vi "Add form to database.vi"(7 "Name":string, 8 "error in (no error)":errorcluster, 11 "Form Server Wrapper in":refnum<class "Form Server Wrapper.lvclass">) -> (0 "error out":errorcluster, 3 "Form Server Wrapper out":refnum<class "Form Server Wrapper.lvclass">)   [LabVIEW 2020, in "Form Server.lvlib" / "Form Server Wrapper.lvclass"]
uses:
  Form Server Wrapper.lvclass
  Form Server Wrapper.lvclass/Form Server Wrapper.ctl
  Form Server Messages Messages/Add Row to Database Msg/Add Row to Database Msg.lvclass/Add Row to Database Msg.ctl
  <vilib>/ActorFramework/Message Enqueuer/Message Enqueuer.lvclass/Message Enqueuer.ctl
  <vilib>/ActorFramework/Message Enqueuer/Enqueue.vi
  Form Server Messages Messages/Add Row to Database Msg/Add Row to Database Msg.lvclass
  C:/Program Files (x86)/National Instruments/LabVIEW 2020/vi.lib/ActorFramework/Message/Message.lvclass
  <vilib>/ActorFramework/Message Priority Queue/Priority Enqueue.vi
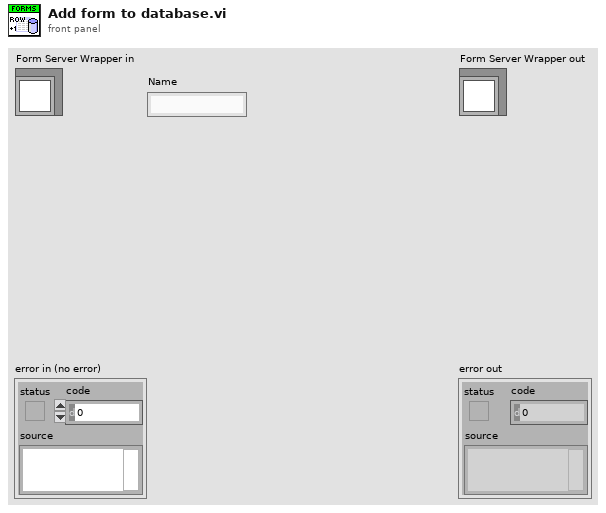
[diagram p1: front panel]
types:
  T1 = typedef "Form Server Interfaces.lvlib/Form ID.ctl" = cluster{"Name":string, "Panel type":string}
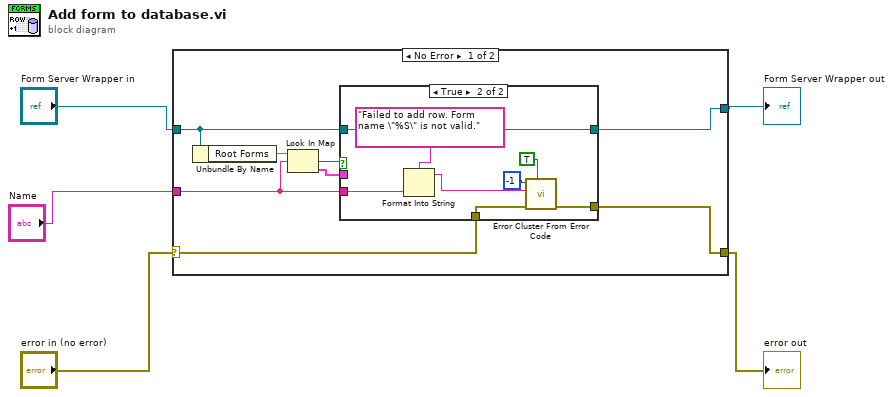
[diagram p0: block diagram]
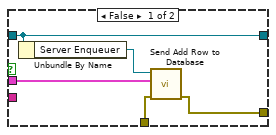
[diagram p2: hidden frame]
diagram:
  n1 = case shown="No Error" "error in (no error)" {
    selector: "error in (no error)" -> [w10 w28]
    tunnel: [w8 w28] -> w2
    tunnel: [w11 w27] -> w4
    tunnel: "Form Server Wrapper in" -> [w6 w27]
    tunnel: "Name" -> [w9 _]
    frame No Error {
      n2 = Unbundle By Name(w6) -> ("Root Forms"=w7:map{string, T1})
      n3 = Look In Map(map=w7, key=w9) -> (key not found?=w13:bool, value=w12:T1)  [unwired: 1 in]
      n4 = case shown="True" w13 {
        tunnel: w12 -> [w15 _]
        tunnel: w6 -> [w18 w23]
        tunnel: [w18 w23] -> w11
        tunnel: w10 -> [w17 w26]
        tunnel: w9 -> [_ w21]
        tunnel: [w16 w19] -> w8
        frame False {
          n5 = Unbundle By Name(w18) -> ("Server Enqueuer"=w14:refnum<class "Message Enqueuer.lvclass">)
          n6 = call "Send Add Row to Database.vi"("error in (no error)"=w17, "Form ID"=w15, "Message Enqueuer"=w14) -> ("error out"=w16:errorcluster)  [unwired: 7 in, 1 out]
        }
        frame True {
          n7 = Format Into String(format string="Failed to add row. Form name \"%S\" is not valid.", w21) -> (resulting string=w20:string)  [unwired: 2 in, 1 out]
          n8 = call <vilib>:"Error Cluster From Error Code.vi"("show call chain? (False)"=TRUE, "error in (no error)"=w26, "error message (\"\")"=w20, "error code (0)"=-1) -> ("error out"=w19:errorcluster)  [unwired: 5 in]
        }
      }
    }
    frame Error {
    }
  }
  "error out" <- w2
  "Form Server Wrapper out" <- w4
